vi "fullCLIENT.vi"() -> ()   [LabVIEW 2023]
uses:
  <vilib>/measure/maspectr.llb/FFT Spectrum (Mag-Phase) for 1 Chan.vi
  <vilib>/measure/NI_MAPro.lvlib
panel:
  in  "Tab Control":enum32{"LOG IN", "HOME PAGE", "HELP"}(tab)
  in  "PORTA":dbl=1500.0 min=1.0 max=65535.0
  in  "SERVER":string="192.168.25.14"
  in  "LOGIN_BUTTON 2":bool
  in  "PASSWORD":string
  out "DIALOG":string
  out "BOOL1":bool
  out "UPDATE 1":string
  out "UPDATE 2":string
  out "BOOL2":bool
  out "BOOL3":bool
  out "PROCESSED SIGNAL":waveform(dbl)(graph)
  out "RAW SIGNAL":waveform(dbl)(graph)
  out "HEART RATE\n [BPM]":dbl
  in  "MIN BPM":dbl=60.0 min=0.0
  in  "MAX BPM":dbl=120.0 min=0.0
  out "WARNING_INDICATOR":bool
  out "WARNING_MESSAGE":string
  in  "SAMPLING FREQUENCY":dbl=1000.0 min=0.0 max=20000.0
  in  "OBSERVATION TIME":dbl=2.0 min=0.0
  in  "MEASURE_BUTTON":bool
  out "PROCESSED FFT-MAG":cluster{"f0":dbl, "df":dbl, "magnitude":dbl[]}(graph)
  # "HEART RATE\nMEASUREMENT"
  # "SIGNAL PARAMETERS"
  # "RESULTS"
  # "THRESHOLD SECTION (HOME PAGE)"
  # "LOGIN SECTION"
  # "VISUAL ANALYSIS  - RAW, PROCESSED, PROCESSED FFT (HOME PAGE)"
  # "1. Use MIN BPM  to set the lower bound of the \n    normal range.\n\n2. Use MAX BPM to set the upper bound of the \n    normal range.\n\nN.B. The default values (i.e. 60-120) represent the\n         clinical reference values."
  # "The VISUAL ANALYSIS SECTION shows the signal processed using the PulseBPM algorithm \nand the FFT spectra of the raw and processed signal."
  # "1. Insert one of the available server.\n\n2. Insert port number or leave default value.\n\n4. Insert the password.\n\n5. Press LOGIN button and wait for \"Connection set\"\n    message."
  # "CREDITS"
  # "MEAS. PARAMETERS (HOME PAGE)"
  # "MEAS. STATUS SECTION (HOME PAGE)"
  # "This work was developed by:\n\n   - Simone Cirnelli, mat.177084\n\n   - Benedetta Dukic, mat.175219\n\n   - Fabrizio Ravelli, mat. 177085\n\n   - Pierfrancesco Romano, mat.177087"
  # "This section provides updates\non the measurement phase such\nas 'Start of Measurement' and\n'End of Measurement'."
  # "1. Select the sampling frequency [sample/s] for the DAQ\n    board.\n\n2. Select the observation time [s] for the DAQ board.\n\n3. Press START button to acquire the signal.\n\nN.B. The values of samp. freq. (fc)  and obs. time (Toss) must \n         be such as to ensure : \n\n                                  fc*Toss < 100000"
  # "RESULT SECTION (HOME PAGE)"
  # "This section provides information on detected\nBPM value."
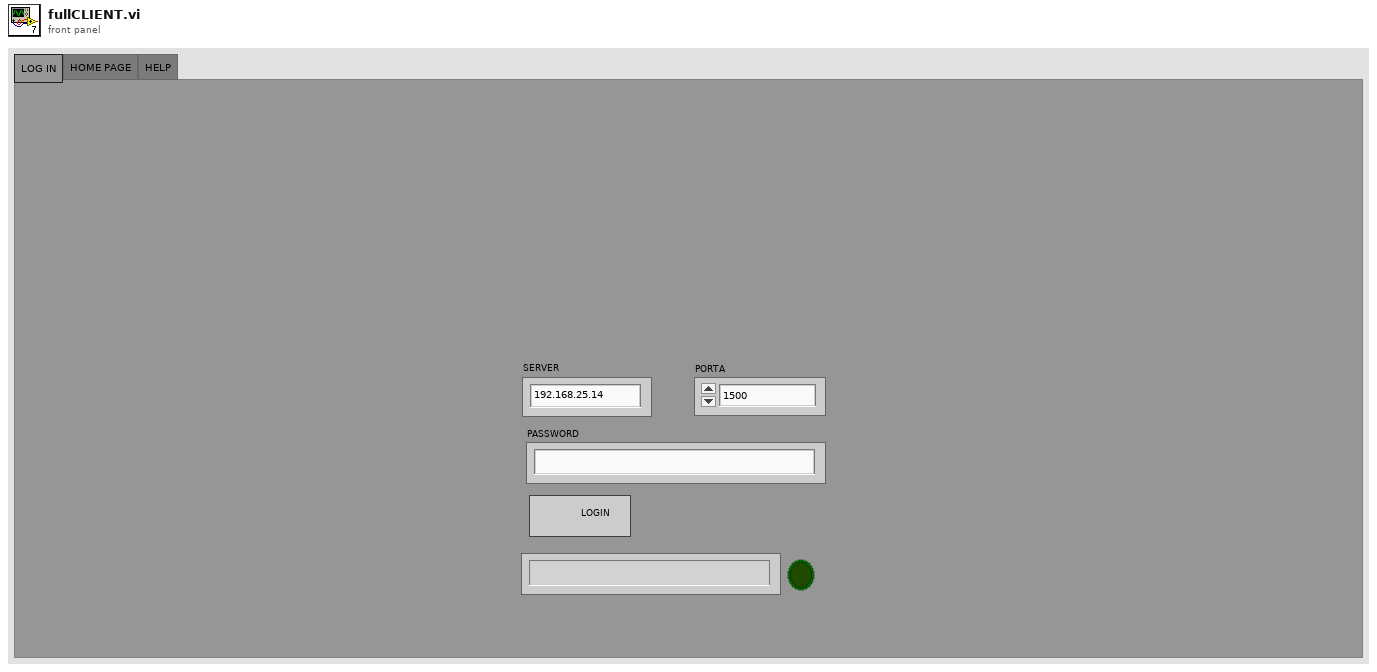
[diagram p1: front panel]
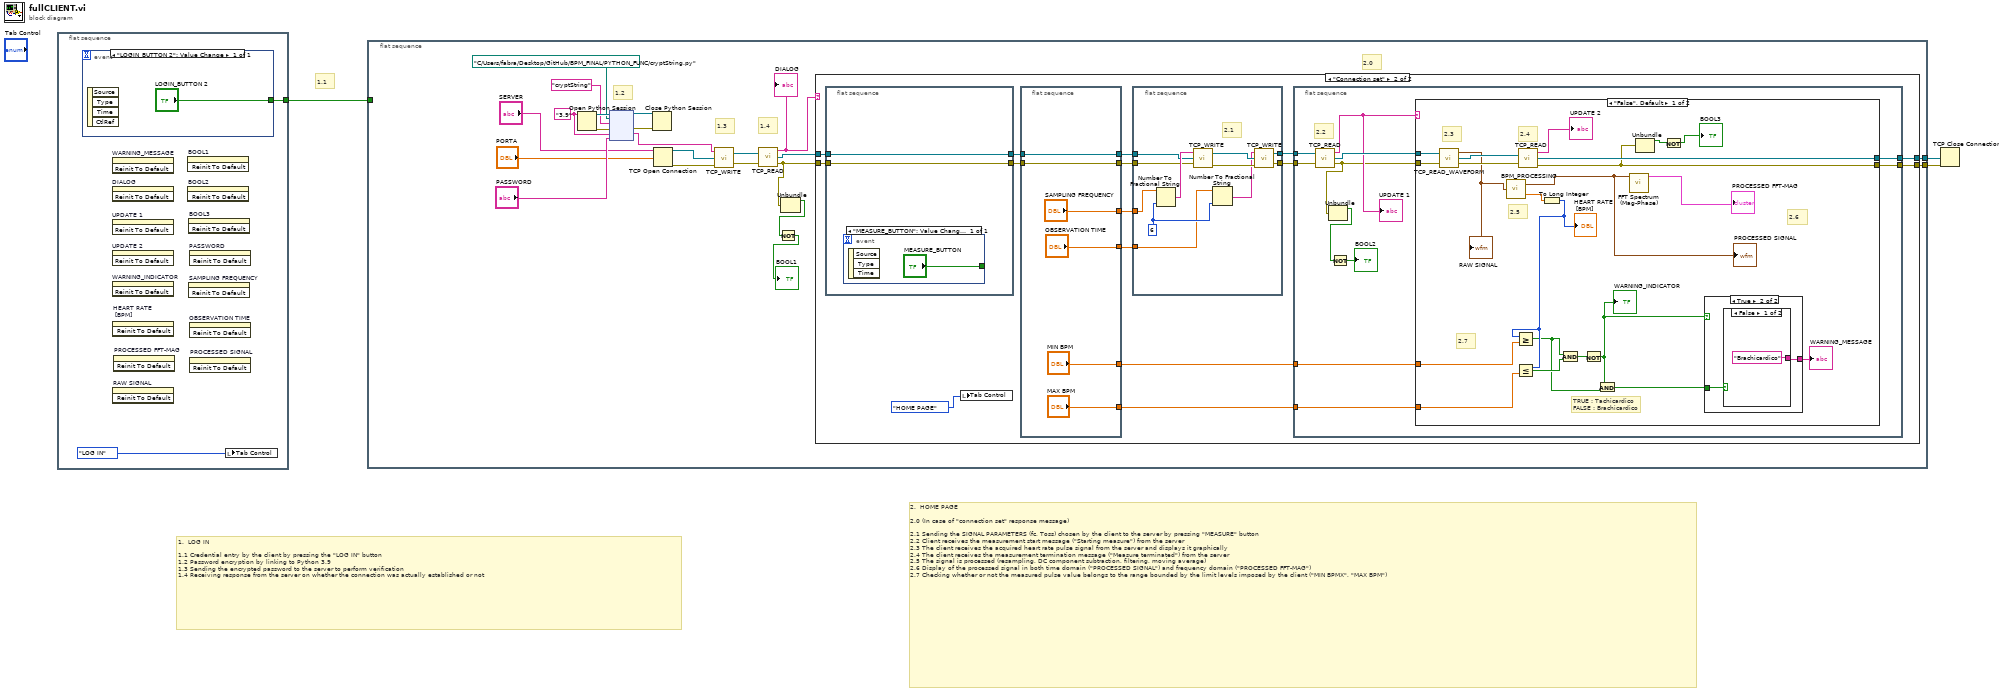
[diagram p0: block diagram]
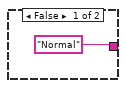
[diagram p3: hidden frame]
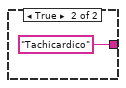
[diagram p4: hidden frame]
diagram:
  # "1.1"
  # "2.  HOME PAGE\n\n2.0 (In case of \"connection set\" response message)\n\n2.1 Sending the SIGNAL PARAMETERS (fc, Toss) chosen by the client to the server by pressing \"MEASURE\" button\n2.2 Client receives the measurement start message (\"Starting measure\") from the server\n2.3 The client receives the acquired heart rate pulse signal from the server and displays it graphically\n2.4 The client receives the measurement termination message (\"Measure terminated\") from the server\n2.5 The signal is processed (resampling, DC component subtraction, filtering, moving average)\n2.6 Display of the processed signal in both time domain (\"PROCESSED SIGNAL\") and frequency domain (\"PROCESSED FFT-MAG\")\n2.7 Checking whether or not the measured pulse value belongs to the range bounded by the limit levels imposed by the client (\"MIN BPMX\", \"MAX BPM\")"
  # "1.  LOG IN \n\n1.1 Credential entry by the client by pressing the \"LOG IN\" button\n1.2 Password encryption by linking to Python 3.9\n1.3 Sending the encrypted password to the server to perform verification\n1.4 Receiving response from the server on whether the connection was actually established or not"
  n1 = flat-sequence {
    tunnel: [w5] -> w3
    frame #0 {
      n2 = event shown="[0] \"LOGIN_BUTTON 2\": Value Change" {
        selector: _ -> [_]
        dyn-events: _ -> [_]
        timeout: _ -> [_]
        tunnel: ["LOGIN_BUTTON 2"] -> w5
        event "LOGIN_BUTTON 2": Value Change {
          n3 = event-data() -> ()  [unwired: 1 in, 4 out]
        }
      }
      n4 = invoke on="WARNING_MESSAGE" class="Str" method="Reinit To Default"() -> ()  [unwired: 3 in, 3 out]
      n5 = invoke on="DIALOG" class="Str" method="Reinit To Default"() -> ()  [unwired: 3 in, 3 out]
      n6 = invoke on="UPDATE 1" class="Str" method="Reinit To Default"() -> ()  [unwired: 3 in, 3 out]
      n7 = invoke on="UPDATE 2" class="Str" method="Reinit To Default"() -> ()  [unwired: 3 in, 3 out]
      n8 = invoke on="WARNING_INDICATOR" class="Bool (strict)" method="Reinit To Default"() -> ()  [unwired: 3 in, 3 out]
      n9 = invoke on="HEART RATE\n [BPM]" class="DigNum (strict)" method="Reinit To Default"() -> ()  [unwired: 3 in, 3 out]
      n10 = invoke on="RAW SIGNAL" class="WFGraph (strict)" method="Reinit To Default"() -> ()  [unwired: 3 in, 3 out]
      n11 = invoke on="PROCESSED FFT-MAG" class="WFGraph (strict)" method="Reinit To Default"() -> ()  [unwired: 3 in, 3 out]
      n12 = invoke on="BOOL1" class="Bool (strict)" method="Reinit To Default"() -> ()  [unwired: 3 in, 3 out]
      n13 = invoke on="BOOL2" class="Bool (strict)" method="Reinit To Default"() -> ()  [unwired: 3 in, 3 out]
      n14 = invoke on="BOOL3" class="Bool (strict)" method="Reinit To Default"() -> ()  [unwired: 3 in, 3 out]
      n15 = invoke on="SAMPLING FREQUENCY" class="DigNum (strict)" method="Reinit To Default"() -> ()  [unwired: 3 in, 3 out]
      n16 = invoke on="PASSWORD" class="Str" method="Reinit To Default"() -> ()  [unwired: 3 in, 3 out]
      n17 = invoke on="OBSERVATION TIME" class="DigNum (strict)" method="Reinit To Default"() -> ()  [unwired: 3 in, 3 out]
      n18 = invoke on="PROCESSED SIGNAL" class="WFGraph (strict)" method="Reinit To Default"() -> ()  [unwired: 3 in, 3 out]
      n19 = local write "Tab Control"(enum32{"LOG IN", "HOME PAGE", "HELP"}."LOG IN" ("Tab Control")) -> ()
    }
  }
  n20 = flat-sequence {
    tunnel: w3 -> [_]
    tunnel: [w23] -> w1
    tunnel: [w22] -> w2
    frame #0 {
      w17 = "3.9" ("Python version")
      # "2.0"
      # "1.4"
      # "1.3"
      # "1.2"
      n21 = Open Python Session(python version=w17) -> (session out=w21:refnum<k35>, error out=w20:errorcluster)  [unwired: 2 in]
      n22 = node(w21, path "C:/Users/fabra/Desktop/GitHub/BPM_FINAL/PYTHON_FUNC/cryptString.py" ("module path"), "cryptString" ("function name"), w20, w17, "PASSWORD") -> (w18:refnum<k35>, w19:errorcluster, w13:string)  [unwired: 1 in, 2 out]
      n23 = Close Python Session(session in=w18, error in=w19) -> ()  [unwired: 1 out]
      n24 = TCP Open Connection(address="SERVER", remote port or service name="PORTA") -> (connection ID=w28:refnum<k5>, error out=w9:errorcluster)  [unwired: 3 in]
      n25 = call "TCP_WRITE.vi"("error in (no error)"=w9, "connection ID"=w28, "data"=w13) -> ("error out"=w26:errorcluster, "connection ID out"=w27:refnum<k5>)
      n26 = call "TCP_READ.vi"("connection ID"=w27, "error in (no error)"=w26) -> ("data"=w24:string, "connection ID out"=w25:refnum<k5>, "error out"=w12:errorcluster)
      "DIALOG" <- w24
      n27 = Unbundle(w12) -> ("status"=w11:bool)  [unwired: 2 out]
      n28 = Not(x=w11) -> (.not. x?=→"BOOL1":bool)
      n29 = case shown="\"Connection set\"" w24 {
        tunnel: w25 -> [w30 w39]
        tunnel: w12 -> [w29 w41]
        tunnel: [w30 w43] -> w23
        tunnel: [w29 w42] -> w22
        frame "False", Default {
        }
        frame "Connection set" {
          n30 = flat-sequence {
            tunnel: w41 -> [w47]
            tunnel: [w47] -> w40
            tunnel: w39 -> [w46]
            tunnel: [w46] -> w38
            frame #0 {
              n31 = event shown="[0] \"MEASURE_BUTTON\": Value Change" {
                selector: _ -> [_]
                dyn-events: _ -> [_]
                timeout: _ -> [_]
                tunnel: ["MEASURE_BUTTON"] -> _
                event "MEASURE_BUTTON": Value Change {
                  n32 = event-data() -> ()  [unwired: 1 in, 3 out]
                }
              }
            }
          }
          n33 = local write "Tab Control"(enum32{"LOG IN", "HOME PAGE", "HELP"}."HOME PAGE" ("Tab Control")) -> ()
          n34 = flat-sequence {
            tunnel: w40 -> [w103]
            tunnel: w38 -> [w102]
            tunnel: ["SAMPLING FREQUENCY"] -> w37
            tunnel: ["OBSERVATION TIME"] -> w36
            tunnel: [w103] -> w35
            tunnel: [w102] -> w34
            tunnel: ["MIN BPM"] -> w33
            tunnel: ["MAX BPM"] -> w32
            frame #0 {
            }
          }
          n35 = flat-sequence {
            tunnel: [w94] -> w45
            tunnel: [w93] -> w44
            tunnel: w37 -> [w92]
            tunnel: w36 -> [w91]
            tunnel: w35 -> [w90]
            tunnel: w34 -> [w89]
            frame #0 {
              w98 = i16 6 ("precision (6)")
              # "2.1"
              n36 = Number To Fractional String(number=w92, precision (6)=w98) -> (F-format string=w99:string)  [unwired: 2 in]
              n37 = call "TCP_WRITE.vi"("error in (no error)"=w90, "connection ID"=w89, "data"=w99) -> ("error out"=w97:errorcluster, "connection ID out"=w96:refnum<k5>)
              n38 = Number To Fractional String(number=w91, precision (6)=w98) -> (F-format string=w95:string)  [unwired: 2 in]
              n39 = call "TCP_WRITE.vi"("error in (no error)"=w97, "connection ID"=w96, "data"=w95) -> ("error out"=w94:errorcluster, "connection ID out"=w93:refnum<k5>)
            }
          }
          n40 = flat-sequence {
            tunnel: w45 -> [w57]
            tunnel: w44 -> [w56]
            tunnel: [w59] -> w43
            tunnel: [w58] -> w42
            tunnel: w33 -> [w53]
            tunnel: w32 -> [w52]
            frame #0 {
              # "2.2"
              n41 = call "TCP_READ.vi"("connection ID"=w56, "error in (no error)"=w57) -> ("data"=w54:string, "connection ID out"=w55:refnum<k5>, "error out"=w51:errorcluster)
              "UPDATE 1" <- w54
              n42 = Unbundle(w51) -> ("status"=w49:bool)  [unwired: 2 out]
              n43 = Not(x=w49) -> (.not. x?=→"BOOL2":bool)
              n44 = case shown="\"False\", Default" w54 {
                tunnel: w51 -> [w80 w88]
                tunnel: w55 -> [w81 w87]
                tunnel: [w76 w87] -> w59
                tunnel: [w65 w88] -> w58
                tunnel: w53 -> [w73 _]
                tunnel: w52 -> [w74 _]
                frame "False", Default {
                  # "2.7"
                  # "2.6"
                  # "2.5"
                  # "2.4"
                  # "2.3"
                  # "TRUE : Tachicardico\nFALSE : Brachicardico"
                  n45 = call "TCP_READ_WAVEFORM.vi"("connection ID"=w81, "error in (no error)"=w80) -> ("waveform"=w62:waveform(dbl), "connection ID out"=w78:refnum<k5>, "error out"=w79:errorcluster)
                  "RAW SIGNAL" <- w62
                  n46 = call "BPM_PROCESSING.vi"("waveform in"=w62) -> ("output waveform"=w61:waveform(dbl), "x*y"=w75:dbl)
                  "PROCESSED SIGNAL" <- w61
                  n47 = call "TCP_READ.vi"("connection ID"=w78, "error in (no error)"=w79) -> ("data"=→"UPDATE 2":string, "connection ID out"=w76:refnum<k5>, "error out"=w65:errorcluster)
                  n48 = To Long Integer(number=w75) -> (32bit integer=w72:i32)
                  "HEART RATE\n [BPM]" <- w72
                  n49 = Greater Or Equal?(x=w72, y=w73) -> (x >= y?=w68:bool)
                  n50 = Less Or Equal?(x=w72, y=w74) -> (x <= y?=w71:bool)
                  n51 = And(x=w68, y=w71) -> (x .and. y?=w70:bool)
                  n52 = Not(x=w70) -> (.not. x?=w67:bool)
                  "WARNING_INDICATOR" <- w67
                  n53 = And(x=w67, y=w68) -> (x .and. y?=w66:bool)
                  n54 = call-poly <vilib>:"FFT Spectrum (Mag-Phase).vi"("time signal"=w61) -> ("magnitude"=→"PROCESSED FFT-MAG":cluster{"f0":dbl, "df":dbl, "magnitude":dbl[]})  [unwired: 6 in, 4 out]
                  n55 = Unbundle(w65) -> ("status"=w64:bool)  [unwired: 2 out]
                  n56 = Not(x=w64) -> (.not. x?=→"BOOL3":bool)
                  n57 = case shown="True" w67 {
                    tunnel: ["Normal" w84] -> w69
                    tunnel: w66 -> [_ w83]
                    frame False {
                    }
                    frame True {
                      n58 = case shown="False" w83 {
                        tunnel: ["Brachicardico" "Tachicardico"] -> w84
                        frame False {
                        }
                        frame True {
                        }
                      }
                    }
                  }
                  "WARNING_MESSAGE" <- w69
                }
                frame "ERROR" {
                }
              }
            }
          }
        }
      }
    }
  }
  n59 = TCP Close Connection(connection ID=w1, error in (no error)=w2) -> ()  [unwired: 1 in, 2 out]
